vi "EEG_acquisition_live.vi"() -> ()   [LabVIEW 2020]
uses:
  <vilib>/Analysis/4window.llb/Hamming Window (DBL).vi
  <vilib>/Analysis/2dsp.llb/Real FFT.vi
  <vilib>/Analysis/1siggen.llb/Ramp Pattern by Samples.vi
  <vilib>/Analysis/4window.llb/AllCosWindow (DBL).vi
  <vilib>/Analysis/NI_AALPro.lvlib
  <vilib>/Analysis/NI_AALBase.lvlib
panel:
  out "Time domain signal":dbl[](graph)
  in  "Press to stop the script":bool
  out "FFT Spectrum":cluster{dbl, dbl}[](graph)
  in  "Alpha low range":dbl
  in  "Alpha high range":dbl
  out "Frequency resolution":dbl
  out "Alpha Spectrum":cluster{"X":dbl, "Y":dbl}[](graph)
  in  "Beta low range":dbl
  in  "Beta high range":dbl
  out "Beta Spectrum":cluster{"X":dbl, "Y":dbl}[](graph)
  out "Gamma Spectrum":cluster{"X":dbl, "Y":dbl}[](graph)
  in  "Gamma low range":dbl
  in  "Gamma high range":dbl
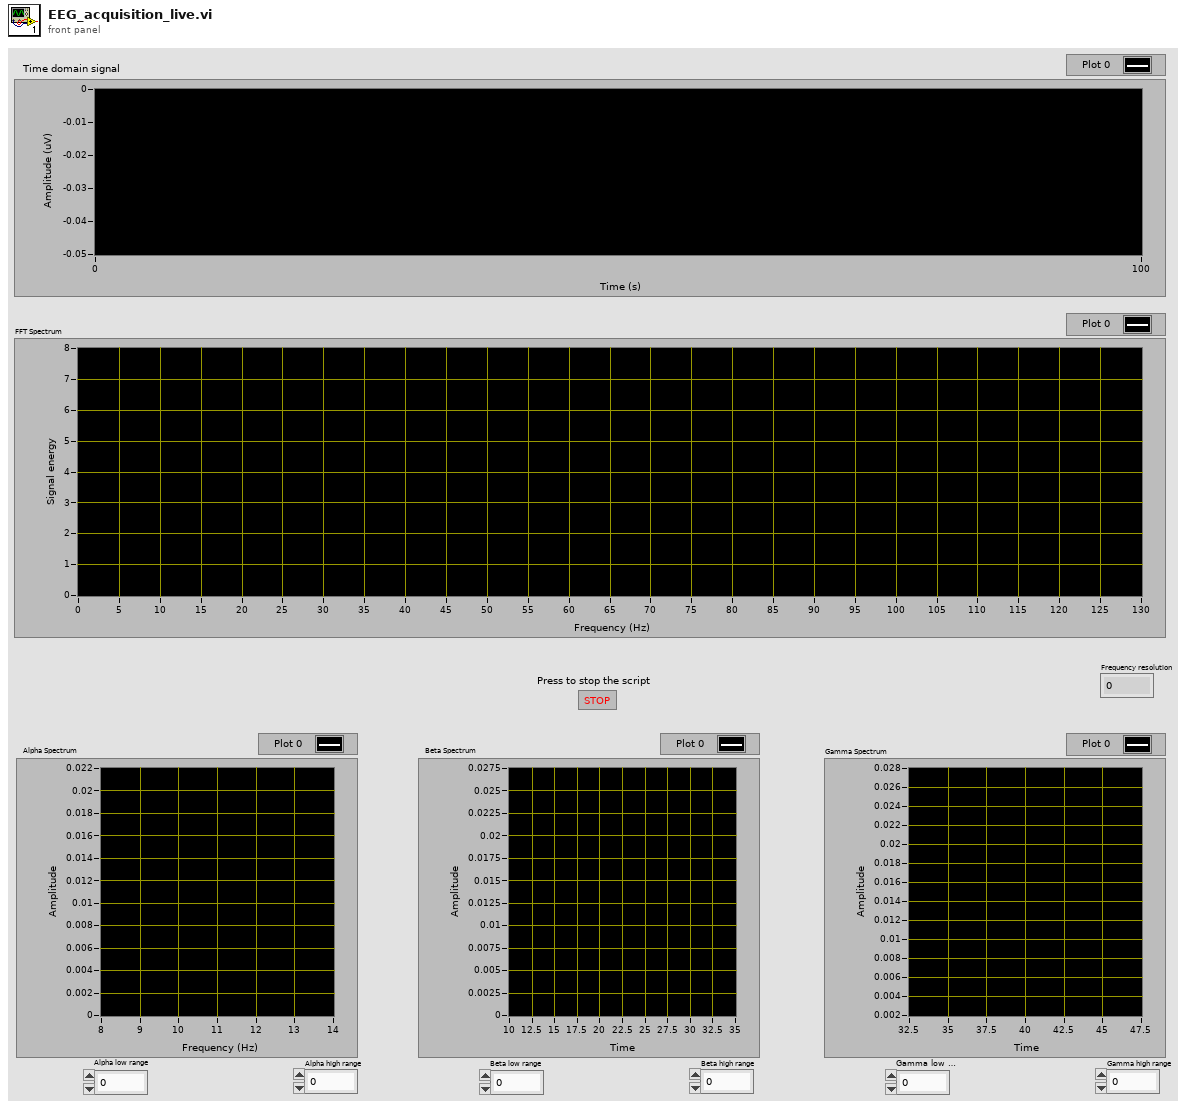
[diagram p1: front panel]
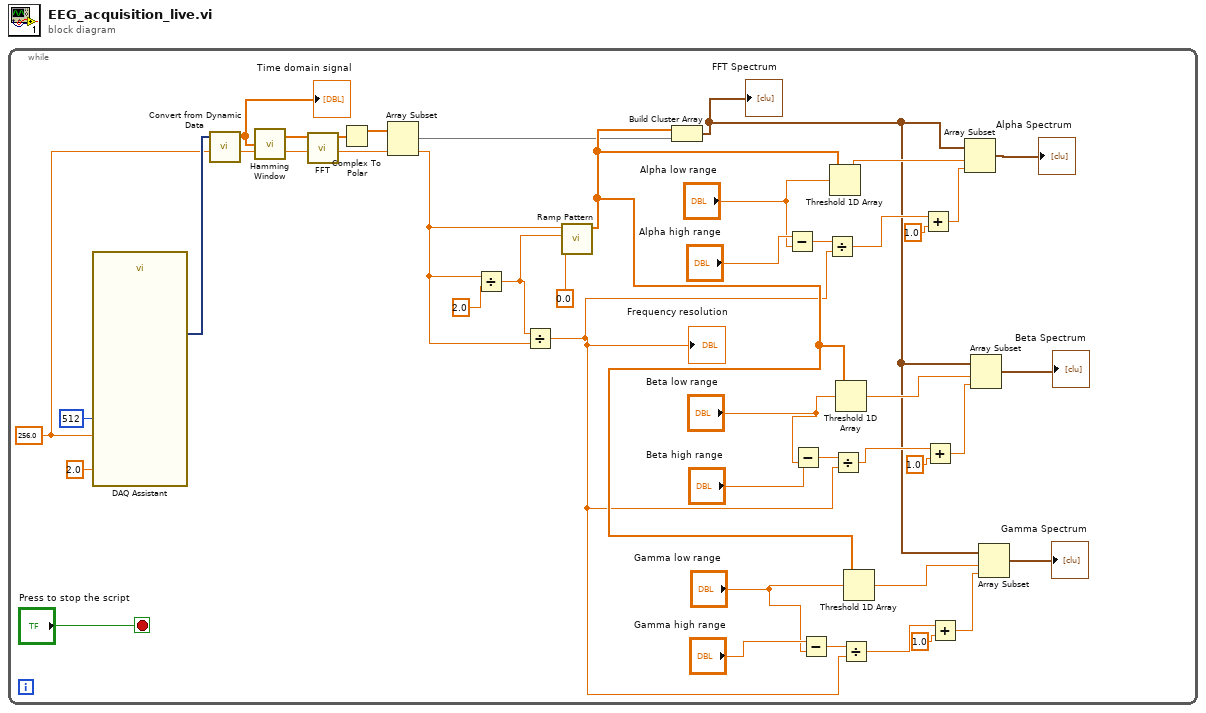
[diagram p0: block diagram]
diagram:
  n1 = while {
    stop <- "Press to stop the script" stop-if-true
    w4 = 256.0 ("sampling rate")
    n2 = call "DAQ Assistant"("rate"=w4, "number of samples"=512, "timeout (s)"=2.0) -> ("data"=w5:dynamicdata)  [unwired: 14 in, 2 out]
    n3 = call "Convert from Dynamic Data"("Dynamic Data Type"=w5) -> ("Array"=w1:dbl[])  [unwired: 3 in]
    "Time domain signal" <- w1
    n4 = call-poly <vilib>:"Hamming Window.vi"("X"=w1) -> ("Windowed X"=w10:dbl[])  [unwired: 1 out]
    n5 = call-poly <vilib>:"FFT.vi"("X"=w10) -> ("FFT {X}"=w40:cdb[])  [unwired: 9 in, 1 out]
    n6 = Complex To Polar(r * e^(i*theta)=w40) -> (r=w37:dbl[])  [unwired: 1 out]
    n7 = Array Subset(array=w37, length=w4) -> (w9:dbl[])  [unwired: 1 in]
    n8 = Divide(x=w4, y=2.0) -> (x/y=w33:dbl)
    n9 = Divide(x=w33, y=w4) -> (x/y=w20:dbl)
    "Frequency resolution" <- w20
    n10 = call-poly <vilib>:"Ramp Pattern.vi"("start"=0.0, "end"=w33, "samples"=w4) -> ("Ramp Pattern"=w22:dbl[])  [unwired: 7 in, 1 out]
    n11 = Build Cluster Array(w22, w9) -> (w8:cluster{dbl, dbl}[])
    "FFT Spectrum" <- w8
    n12 = Subtract(x="Alpha high range", y="Alpha low range") -> (x-y=w32:dbl)
    n13 = Subtract(x="Beta high range", y="Beta low range") -> (x-y=w29:dbl)
    n14 = Subtract(x="Gamma high range", y="Gamma low range") -> (x-y=w24:dbl)
    n15 = Divide(x=w32, y=w20) -> (x/y=w11:dbl)
    n16 = Threshold 1D Array(2:"Alpha low range", 3:w22) -> (0:w36:dbl)  [unwired: 1 in]
    n17 = Divide(x=w29, y=w20) -> (x/y=w15:dbl)
    n18 = Threshold 1D Array(2:"Beta low range", 3:w22) -> (0:w28:dbl)  [unwired: 1 in]
    n19 = Divide(x=w24, y=w20) -> (x/y=w19:dbl)
    n20 = Threshold 1D Array(2:"Gamma low range", 3:w22) -> (0:w23:dbl)  [unwired: 1 in]
    n21 = Add(x=w11, y=1.0) -> (x+y=w12:dbl)
    n22 = Add(x=w15, y=1.0) -> (x+y=w14:dbl)
    n23 = Add(x=w19, y=1.0) -> (x+y=w18:dbl)
    n24 = Array Subset(array=w8, index=w36, length=w12) -> (→"Alpha Spectrum":cluster{dbl, dbl}[])
    n25 = Array Subset(array=w8, index=w28, length=w14) -> (→"Beta Spectrum":cluster{dbl, dbl}[])
    n26 = Array Subset(array=w8, index=w23, length=w18) -> (→"Gamma Spectrum":cluster{dbl, dbl}[])
  }
